vi "GetServiceRequestStatus.vi"(0 "VISA resource name":refnum<visa-resource-name>, 11 "error in":errorcluster) -> (4 "VISA resource name out":refnum<visa-resource-name>, 6 "Service request status string":string, 8 "Service request status":i32, 10 "Binary String":string, 15 "error out":errorcluster)   [LabVIEW 2023, in "Thermotron 8800.lvlib"]
doc: "SRQB\nCommand name: Send service request status byte\nCommand type: System status\nDescription: The 8800 returns the same data that a GPIB serial poll would return. The events, which set the associated bits in the response data, must be enabled in the SRQ mask and are loaded using the SRQM command. The bits are defined as follows:\nBit # Definition \n0 Change in state\n1 Change in alarm status \n2 End of interval \n3 Match interval \n4 End of program\n5 Error\n6 Reserved by GPIB (RSV)\n7 Power on reset\nSyntax: SRQB?\nData type: Coded integer\nQuery example: SRQB?\n8800 response: 65 = 01000001\nbit 7 bit 6 bit 5 bit 4 bit 3 bit 2 bit 1 bit 0\n 0 1 0 0 0 0 0 1\n(This response indicates state change + RSV.)"
uses:
  Thermotron 8800.lvlib
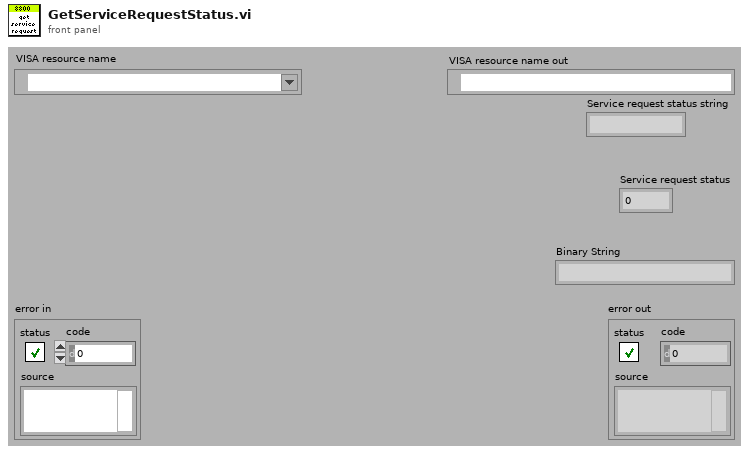
[diagram p1: front panel]
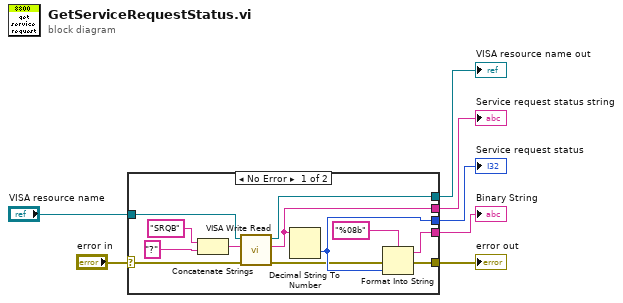
[diagram p0: block diagram]
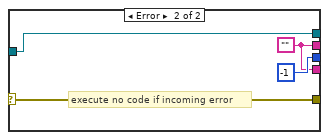
[diagram p2: hidden frame]
diagram:
  n1 = case shown="No Error" "error in" {
    selector: "error in" -> [w18 w23]
    tunnel: [w8 w23] -> w5
    tunnel: [w17 w22] -> w4
    tunnel: "VISA resource name" -> [w15 w22]
    tunnel: [w13 w20] -> w1
    tunnel: [w11 -1] -> w2
    tunnel: [w10 w20] -> w3
    frame No Error {
      n2 = Concatenate Strings("SRQB" ("8800 Command"), "?" ("8800 Command")) -> (w19:string)
      n3 = call "VISA Write Read.vi"("error in (no error)"=w18, "8800 Command"=w19, "VISA Refnum in"=w15) -> ("error out"=w9:errorcluster, "read buffer"=w13:string, "VISA Refnum out"=w17:refnum<visa-resource-name>)  [unwired: 6 in]
      n4 = Decimal String To Number(string=w13) -> (number=w11:i32)  [unwired: 2 in, 1 out]
      n5 = Format Into String(format string="%08b", error in=w9, w11) -> (resulting string=w10:string, error out=w8:errorcluster)  [unwired: 1 in]
    }
    frame Error {
      w20 = ""
      # "execute no code if incoming error"
    }
  }
  "VISA resource name out" <- w4
  "error out" <- w5
  "Binary String" <- w3
  "Service request status" <- w2
  "Service request status string" <- w1
